vi "Update Status.vi"(8 "error in (no error)":errorcluster, 10 "Status Message":string, 11 "Splash Screen in":refnum<class "Splash Screen.lvclass">) -> (0 "error out":errorcluster, 3 "Splash Screen out":refnum<class "Splash Screen.lvclass">)   [LabVIEW 2015, in "Splash Screen.lvlib" / "Splash Screen.lvclass"]
uses:
  Splash Screen.lvclass
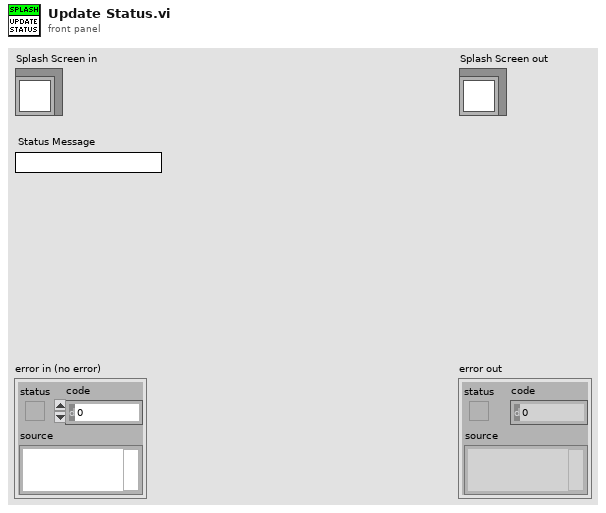
[diagram p1: front panel]
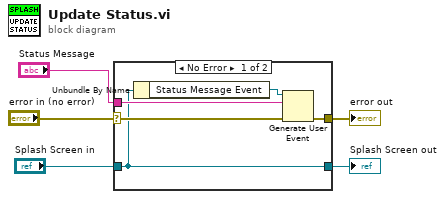
[diagram p0: block diagram]
diagram:
  n1 = case shown="No Error" "error in (no error)" {
    selector: "error in (no error)" -> [w8 w12]
    tunnel: [w7 w12] -> w4
    tunnel: [w6 w11] -> w2
    tunnel: "Splash Screen in" -> [w6 w11]
    tunnel: "Status Message" -> [w9 _]
    frame No Error {
      n2 = Unbundle By Name(w6) -> ("Status Message Event"=w10:refnum<user-event>)
      n3 = Generate User Event(user event=w10, event data cluster=w9, error in=w8) -> (error out=w7:errorcluster)  [unwired: 1 in, 1 out]
    }
    frame Error {
    }
  }
  "error out" <- w4
  "Splash Screen out" <- w2
